vi "ex8-9.vi"   [LabVIEW 2009]
uses:
  <vilib>/NXT/Block Support/NXT_MessageMailbox.ctl
  <vilib>/NXT/Dual Mode Library/Display/drawText.vi
  <vilib>/NXT/Dual Mode Library/BT/BlueTooth_Read_string.vi
types:
  T1 = typedef "NXT_MessageMailbox.ctl" = u8
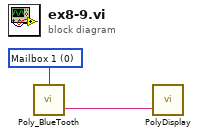
[diagram p0: block diagram]
diagram:
  w2 = T1 0 items=["Mailbox 1", "Mailbox 2", "Mailbox 3", "Mailbox 4", "Mailbox 5", "Mailbox 6", "Mailbox 7", "Mailbox 8", "Mailbox 9", "Mailbox 10"] ("Mailbox")
  n1 = call-poly <vilib>:"Poly_BlueTooth.vi"("Mailbox"=w2) -> ("Message"=w1:string)  [unwired: 2 in, 1 out]
  n2 = call-poly <vilib>:"PolyDisplay.vi"("Text"=w1) -> ()  [unwired: 3 in, 1 out]
